vi "MotorControlMina4 with Joystick control3.vi"() -> ()   [LabVIEW 2014]
uses:
  <vilib>/Utility/inputDevices.llb/joystickAcquire.vi
  <vilib>/Utility/inputDevices.llb/closeJoystick.vi
panel:
  out "joystick info":T1(array[cluster])
  in  "Stop":bool
  out "InstrumentMode":T2(ring)=enum."Shutdown"
  in  "XMotorRef":refnum<k7>(container)
  in  "YMotorRef":refnum<k7>(container)
  in  "ZMotorRef":refnum<k7>(container)
  out "JoystOffset":T3={"XOffset"=-99999, "YOffset"=-99999, "ZOffset"=-99999}
  out "RelJoyPos":T4
  in  "InterfaceSelector":T5(tab)
  in  "GoToTopDisp":bool
  in  "GoToBottDisp":bool
  in  "GoToExpLoc":bool
  in  "SaveTopDisp":bool
  in  "SaveBottDisp":bool
  in  "SaveExpLoc":bool
  out "Top Dispenser":T6={"X Pos (mm)"=0.5532008, "Y Pos (mm)"=0.030929338, "Z Pos (mm)"=0.77973413} {"Y Pos (mm)" format="%.3f"; "Z Pos (mm)" format="%.3f"; "X Pos (mm)" format="%.3f"}
  out "Bottom Dispenser":T6={"X Pos (mm)"=0.600309, "Y Pos (mm)"=-1.1540928, "Z Pos (mm)"=0.7938141} {"Y Pos (mm)" format="%.3f"; "Z Pos (mm)" format="%.3f"; "X Pos (mm)" format="%.3f"}
  out "Experiment Region":T6={"X Pos (mm)"=1.4278219, "Y Pos (mm)"=-0.74810517, "Z Pos (mm)"=0.7938141} {"Y Pos (mm)" format="%.3f"; "Z Pos (mm)" format="%.3f"; "X Pos (mm)" format="%.3f"}
  in  "PreviewPanel":T7(tab)
  in  "Z Motor Settings":T8={"Joyst Min Signal"=10.0, "Joyst Max Signal"=30000.0, "Vmax (mm/s)"=0.005, "Acc (mm/s/s)"=0.2, "+ JoystDirection"=2, "- JoystDirection"=1} {"Acc (mm/s/s)" format="%#.3f"; "Vmax (mm/s)" format="%#.3f"}
  in  "Y Motor Settings":T8={"Joyst Min Signal"=10.0, "Joyst Max Signal"=20000.0, "Vmax (mm/s)"=0.03, "Acc (mm/s/s)"=0.5, "+ JoystDirection"=1, "- JoystDirection"=2} {"Acc (mm/s/s)" format="%#.3f"; "Vmax (mm/s)" format="%#.3f"}
  in  "X Motor Settings":T8={"Joyst Min Signal"=10.0, "Joyst Max Signal"=20000.0, "Vmax (mm/s)"=0.03, "Acc (mm/s/s)"=0.5, "+ JoystDirection"=2, "- JoystDirection"=1} {"Acc (mm/s/s)" format="%#.3f"; "Vmax (mm/s)" format="%#.3f"}
  in  "Motor Cruise Param":T9={"X Acc (mm/s^2)"=0.3, "X Vmax (mm/s)"=0.3, "Y Acc (mm/s^2)"=0.3, "Y Vmax (mm/s)"=0.3, "Z Acc (mm/s^2)"=0.1, "Z Vmax (mm/s)"=0.1}
  in  "Motor Limits":T10={"XMin"=-0.8, "XMax"=3.0, "YMin"=-2.0, "YMax"=2.0, "ZMin"=0.0, "ZMax"=2.0}
  in  "Steerable Mirror Calibration":T11={"Hor. Scaling (nm/V)"=760.0, "Vert. Scaling (nm/V)"=760.0, "Hor. Mirr. Offset (V)"=0.0, "Vert. Mirr. Offset (V)"=0.0}
  in  "Steerable \nTrap\n(F12)":bool
  in  "Fixed\nTrap\n(F11)":bool
  in  "Align Traps Vertically":bool
  in  "MaxHorizontalTrapSeparation":bool
  out "X Motor State":T12={"Direction"=0, "Vel (mm/s)"=0.0, "IsActive?"=FALSE, "Pos (mm)"=-0.2957381} {"Pos (mm)" format="%#.3f"; "Vel (mm/s)" format="%#.4f"}
  out "Y Motor State":T12={"Direction"=0, "Vel (mm/s)"=0.0, "IsActive?"=FALSE, "Pos (mm)"=0.016441232} {"Pos (mm)" format="%#.3f"; "Vel (mm/s)" format="%#.4f"}
  out "Z Motor State":T12={"Direction"=0, "Vel (mm/s)"=0.0, "IsActive?"=FALSE, "Pos (mm)"=-0.26253498} {"Pos (mm)" format="%#.3f"; "Vel (mm/s)" format="%#.4f"}
  out "Move Z":bool
  out "Move XY":bool
  in  "MotorLoopDelay":u32=100
  in  "StopPassiveMode":bool caption="stop"
  in  "PMVertSlider(V)":dbl(slide)=0.005145263671875 scale=0.0..10.0 scale format="%#_3f"
  in  "PMHorizSlider(V)":dbl(slide)=0.0045623779296875 scale=2.0..10.0
  out "IsPassiveModeActive?":bool caption="stop"
  out "Force TrapA":cluster{"x":dbl[], "y":dbl[]}[](graph)
  out "Noise-Ext":cluster{"x":dbl[], "y":dbl[]}[](graph)
  out "Force TrapB":cluster{"x":dbl[], "y":dbl[]}[](graph)
  out "IsOffsetModeActive?":bool caption="stop"
  in  "StopOffset":bool caption="stop"
  out "IsForceExtActive?":bool=TRUE
  in  "StopForceExtension":bool caption="stop"
  # "ClpXP Optical Tweezers"
  # "Chamber Locations"
  # "Need a Button Here that would read the \nNormalized Offset and save it"
  # "Off"
  # "On"
  # "Off"
  # "On"
  # "Thorlabs Motor Status"
  # "Passive Mode"
  # "when I switch tabs from the passive mode to basic mode, the recording doesn't stop"
  # "The sliders don't do anything in passive mode, fix it"
  # "Whenever I click on Ackquire Offset, it goes back to the basic operation, then I have to ckick again"
  # "Trap Motion Control"
  # "Steerable Mirror Info"
  # "Zero-Force Offset Mode"
  # "High Frequency Data Acquisition"
  # "Adjust the length of acquisition time"
  # "Force-Extension Mode"
  # "Y"
  # "+"
  # "X"
  # "-"
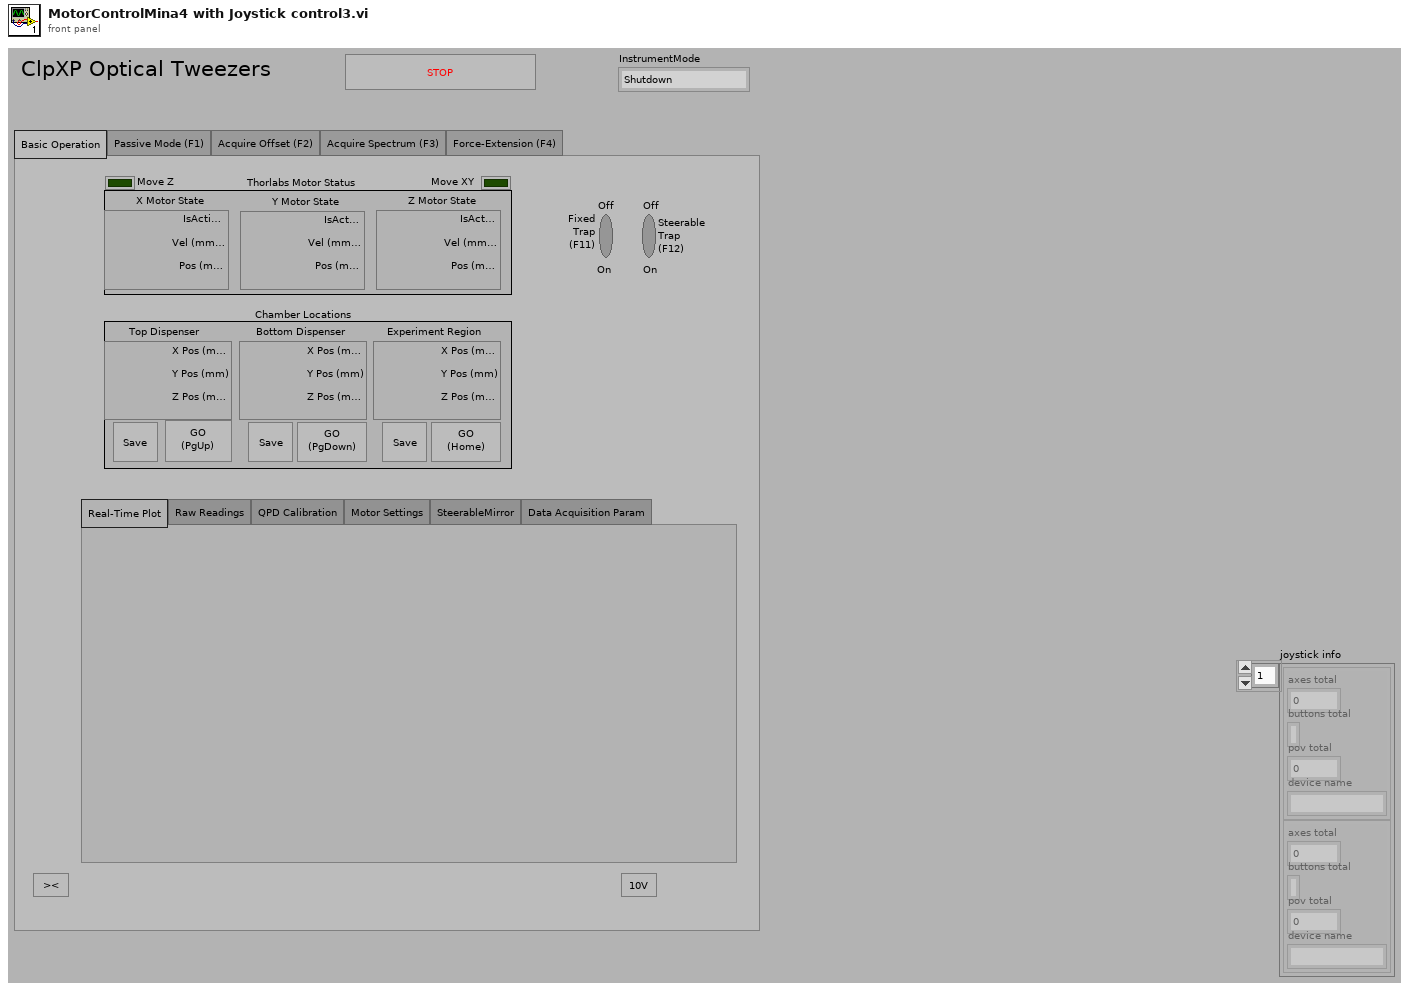
[diagram p1: front panel]
types:
  T1 = cluster{"axes total":u32, "buttons total":u32, "pov total":u32, "device name":string}[]
  T2 = enum16{"InitializeJoystick", "InitializeMotors", "BasicMode", "PassiveMode", "AcquireOffsetMode", "AcquireSpectrumMode", "Force-ExtensionMode", "Shutdown"}
  T3 = cluster{"XOffset":i32, "YOffset":i32, "ZOffset":i32}
  T4 = cluster{"XRelPos":i32, "YRelPos":i32, "ZRelPos":i32}
  T5 = enum32{"Basic Operation", "Passive Mode (F1)", "Acquire Offset (F2)", "Acquire Spectrum (F3)", "Force-Extension (F4)"}
  T6 = cluster{"X Pos (mm)":sgl, "Y Pos (mm)":sgl, "Z Pos (mm)":sgl}
  T7 = enum32{"Real-Time Plot", "Raw Readings", "QPD Calibration", "Motor Settings", "SteerableMirror", "Data Acquisition Param"}
  T8 = cluster{"Joyst Min Signal":dbl, "Joyst Max Signal":dbl, "Vmax (mm/s)":sgl, "Acc (mm/s/s)":sgl, "+ JoystDirection":i32, "- JoystDirection":i32}
  T9 = cluster{"X Acc (mm/s^2)":sgl, "X Vmax (mm/s)":sgl, "Y Acc (mm/s^2)":sgl, "Y Vmax (mm/s)":sgl, "Z Acc (mm/s^2)":sgl, "Z Vmax (mm/s)":sgl}
  T10 = cluster{"XMin":sgl, "XMax":sgl, "YMin":sgl, "YMax":sgl, "ZMin":sgl, "ZMax":sgl}
  T11 = cluster{"Hor. Scaling (nm/V)":dbl, "Vert. Scaling (nm/V)":dbl, "Hor. Mirr. Offset (V)":dbl, "Vert. Mirr. Offset (V)":dbl}
  T12 = cluster{"Direction":i32, "Vel (mm/s)":sgl, "IsActive?":bool, "Pos (mm)":sgl}
  T13 = cluster{"XMotorRef":refnum<k7>, "YMotorRef":refnum<k7>, "ZMotorRef":refnum<k7>}
  T14 = cluster{"Motor Reference":refnum<k7>, "Motor Reference":refnum<k7>, "Motor Reference":refnum<k7>}
  T15 = cluster{"X axis":i32, "Y axis":i32, "Z axis":i32, "X axis rotation":i32, "Y axis rotation":i32, "Z axis rotation":i32, "U axis":i32, "V axis":i32}
  T16 = cluster{"button 1":bool, "button 2":bool, "button 3":bool, "button 4":bool, "button 5":bool, "button 6":bool, "button 7":bool, "button 8":bool, "button 9":bool, "button 10":bool, "button 11":bool, "button 12":bool, "button 13":bool, "button 14":bool, "button 15":bool, "button 16":bool, "button 17":bool, "button 18":bool, "button 19":bool, "button 20":bool, "button 21":bool, "button 22":bool, "button 23":bool, "button 24":bool, "button 25":bool, "button 26":bool, "button 27":bool, "button 28":bool, "button 29":bool, "button 30":bool, "button 31":bool, "button 32":bool}
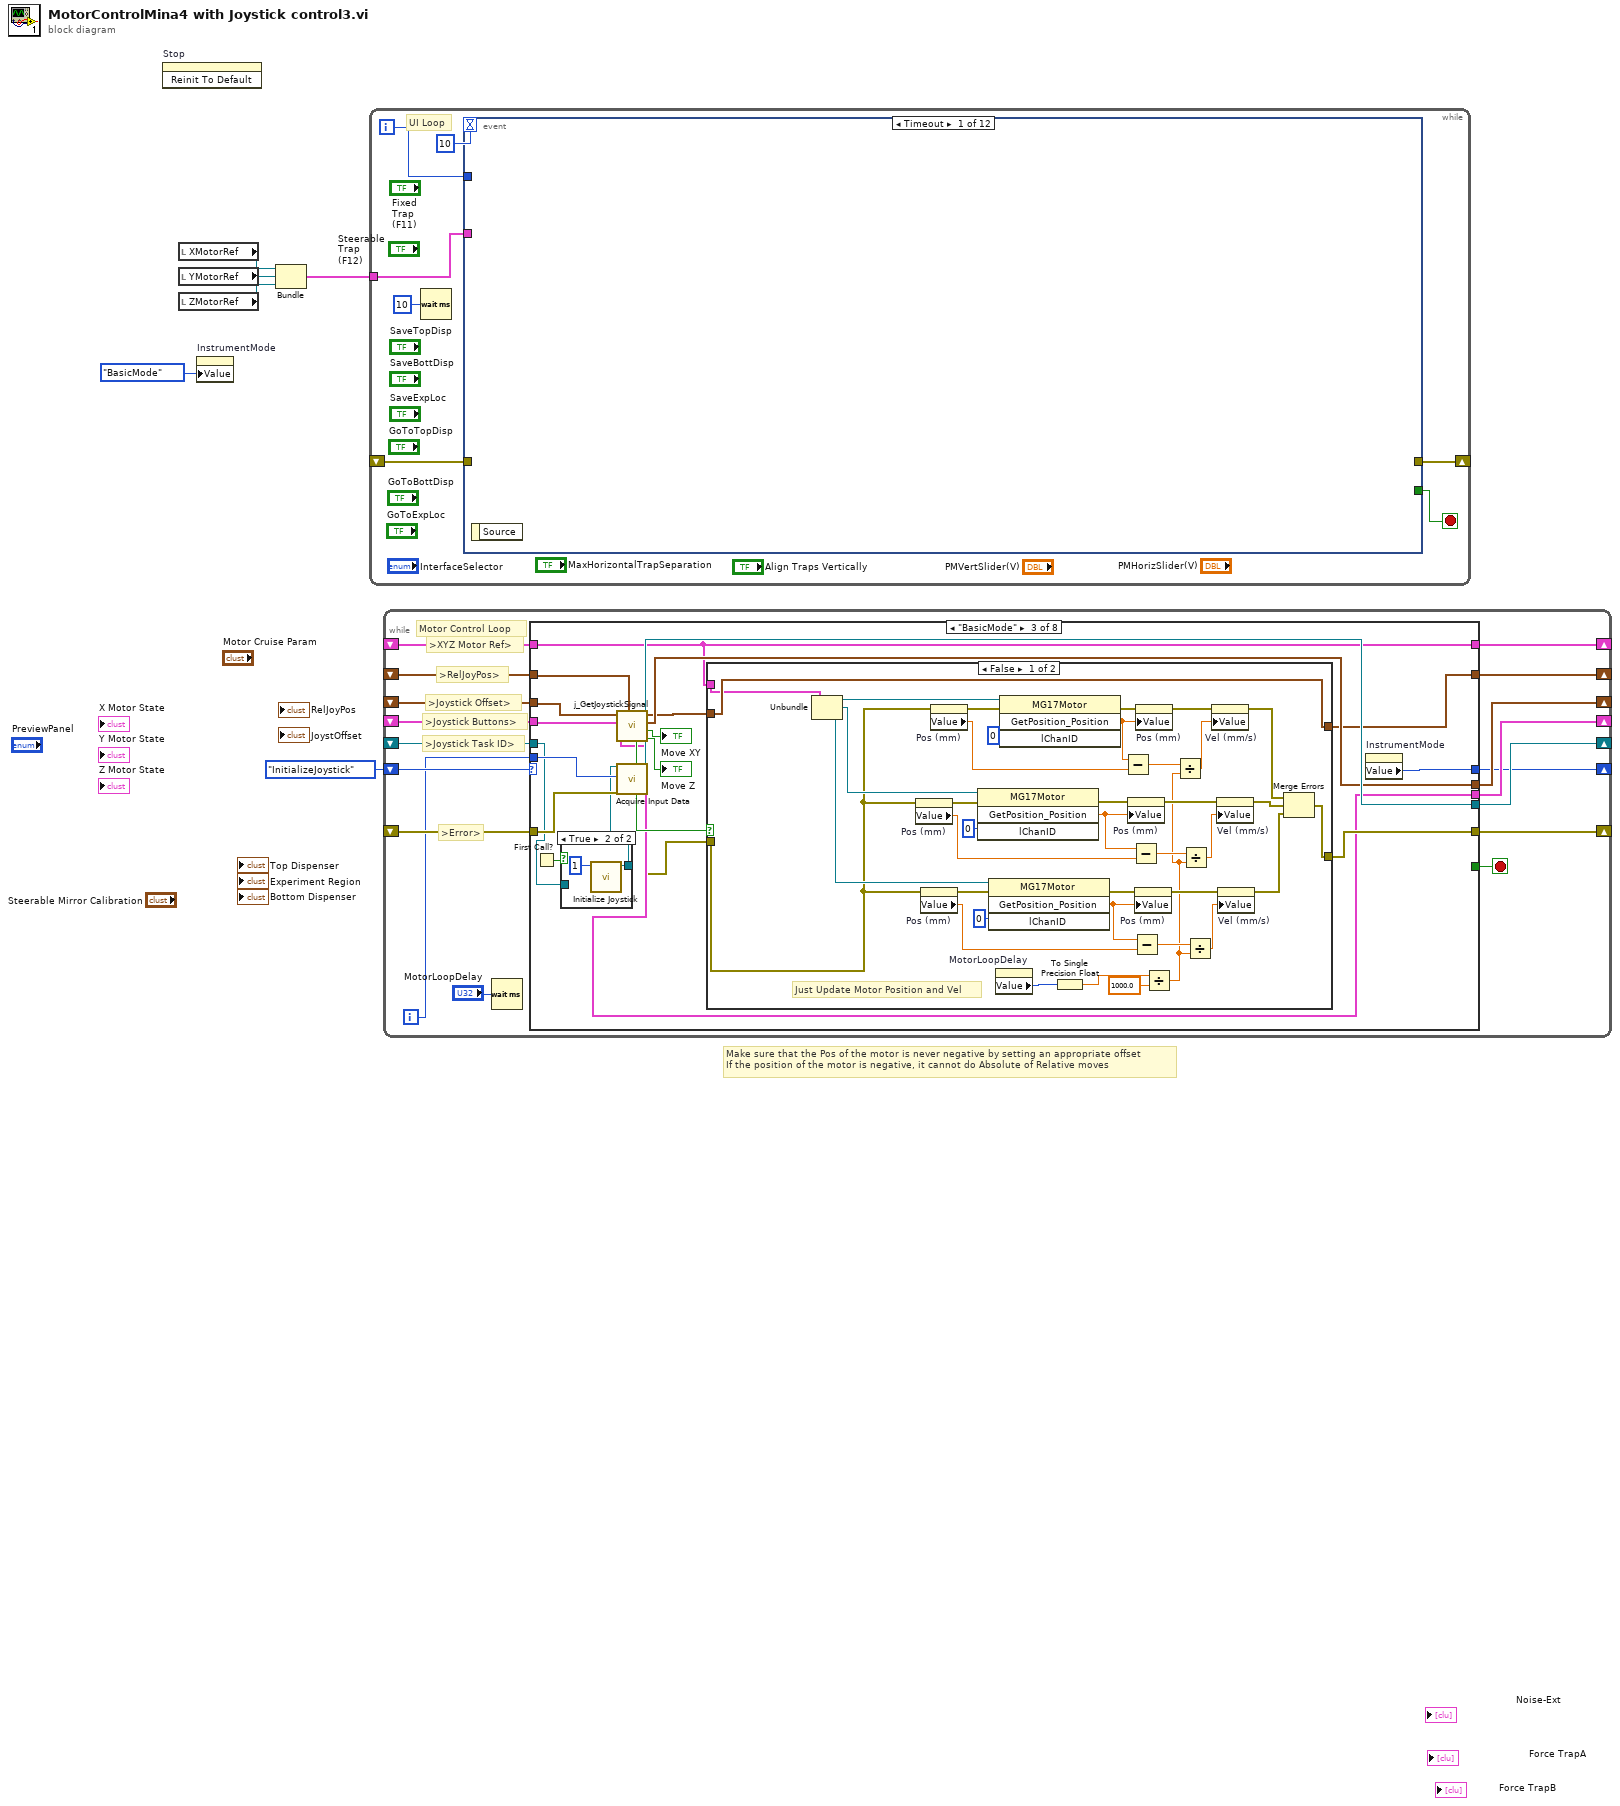
[diagram p0: block diagram]
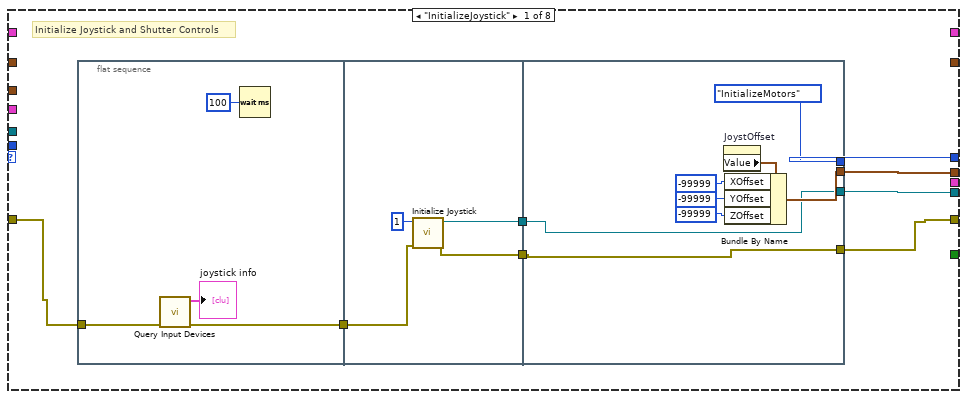
[diagram p2: hidden frame]
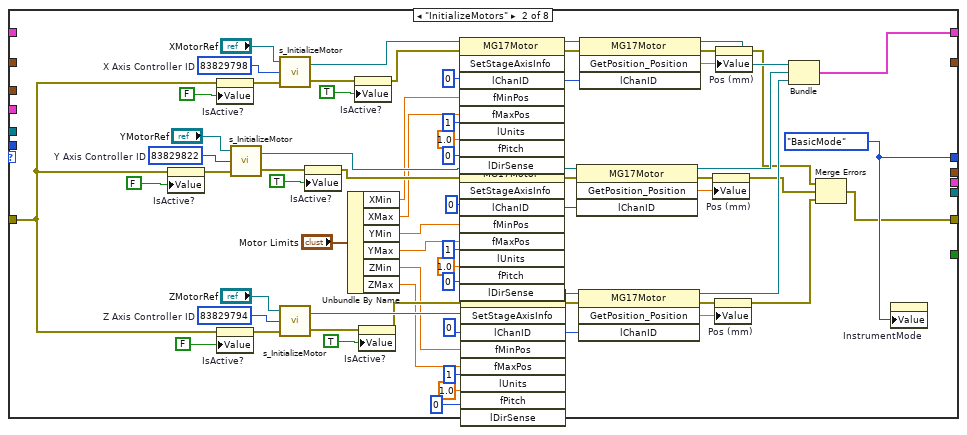
[diagram p3: hidden frame]
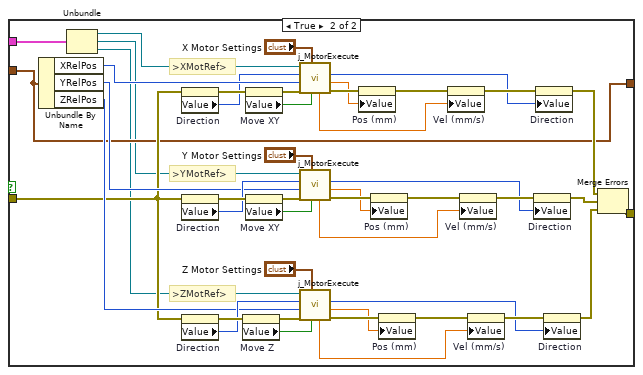
[diagram p5: hidden frame]
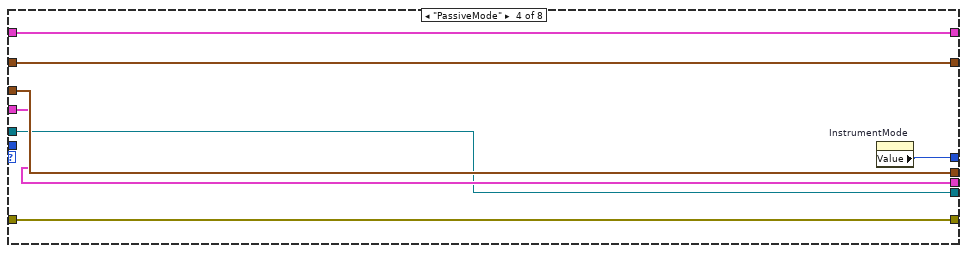
[diagram p6: hidden frame]
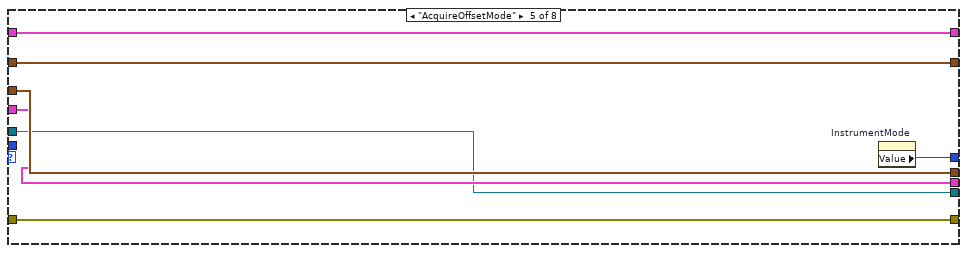
[diagram p7: hidden frame]
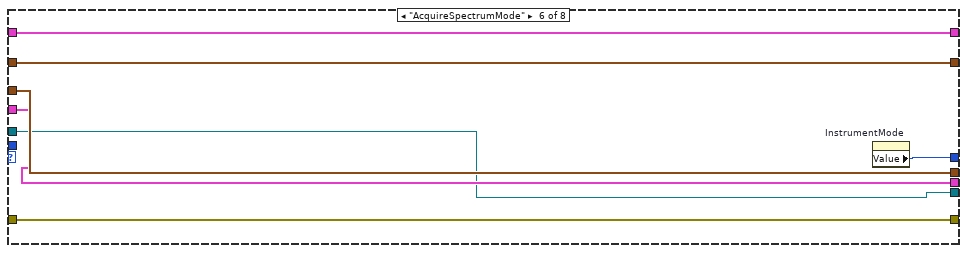
[diagram p8: hidden frame]
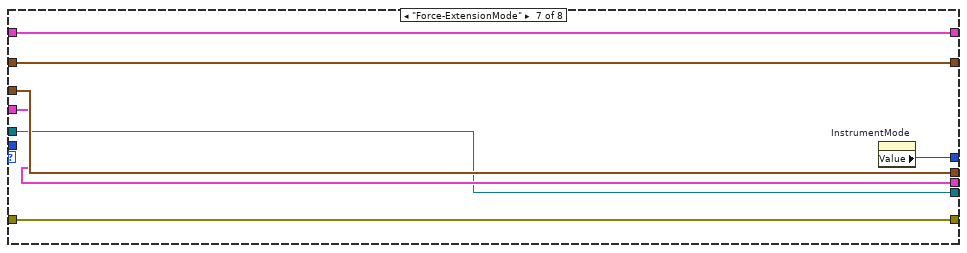
[diagram p9: hidden frame]
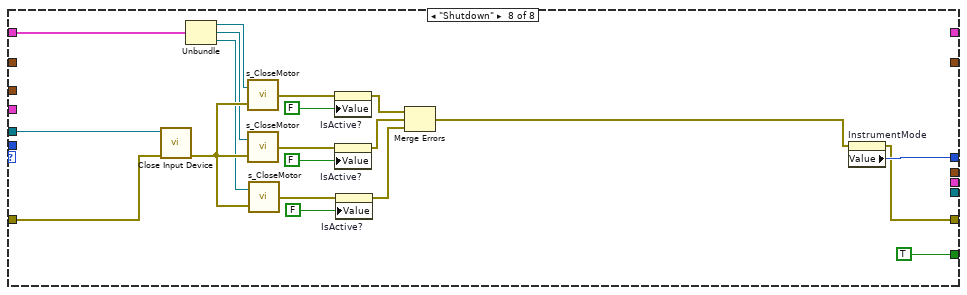
[diagram p10: hidden frame]
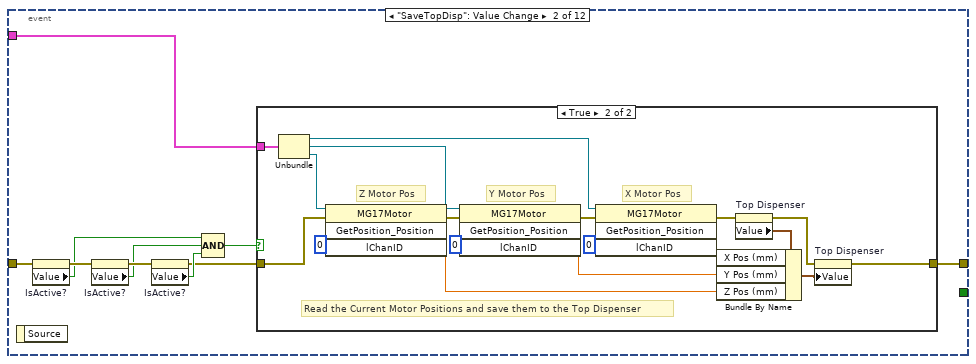
[diagram p11: hidden frame]
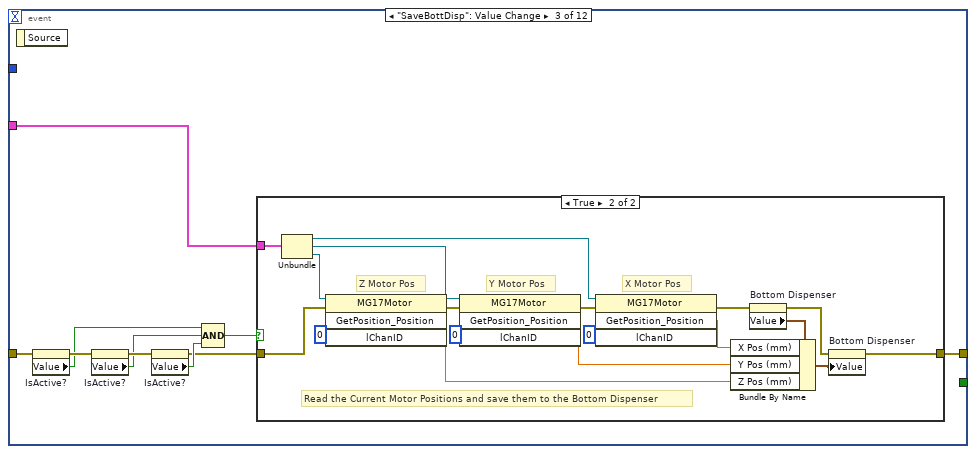
[diagram p13: hidden frame]
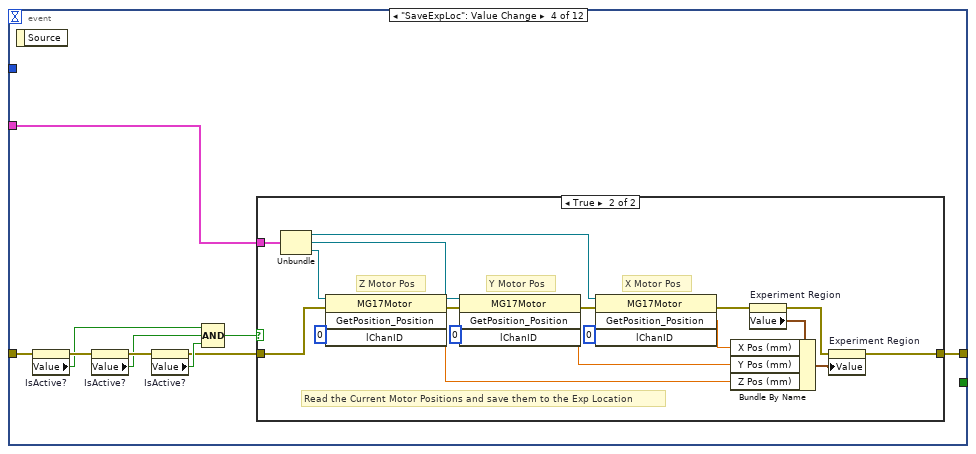
[diagram p15: hidden frame]
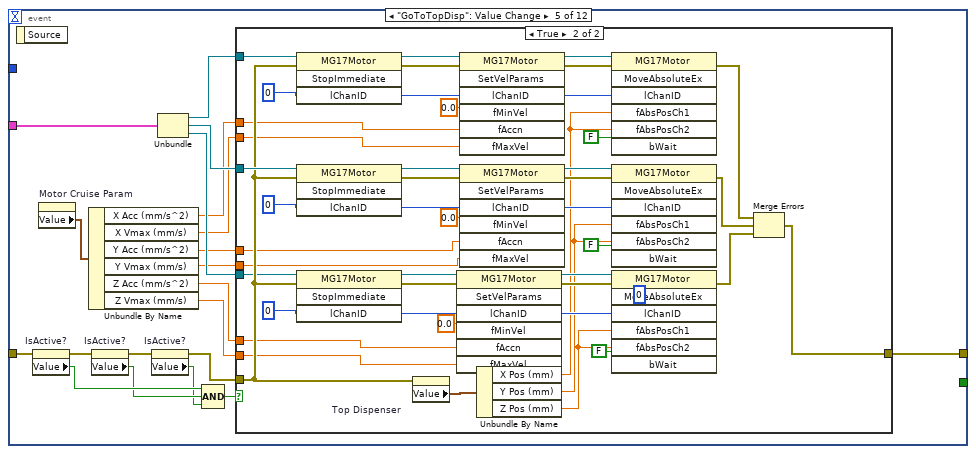
[diagram p17: hidden frame]
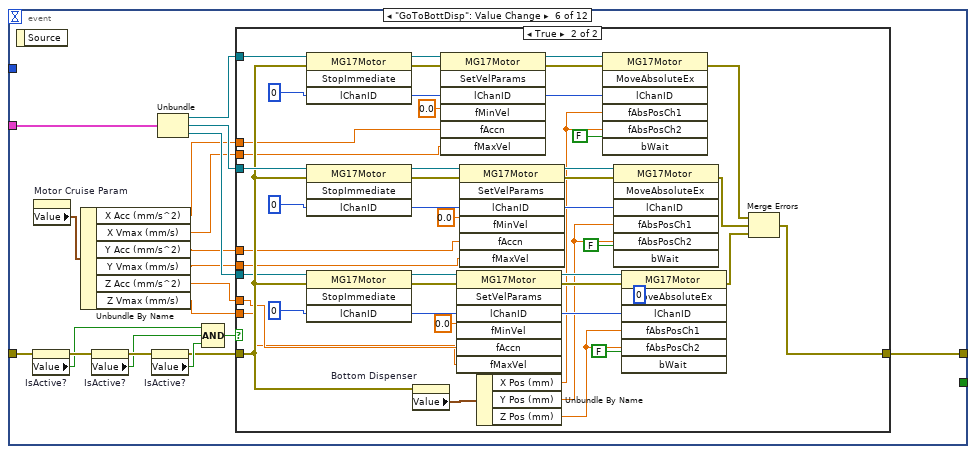
[diagram p19: hidden frame]
diagram:
  # "Make sure that the Pos of the motor is never negative by setting an appropriate offset\nIf the position of the motor is negative, it cannot do Absolute of Relative moves"
  n1 = invoke on="Stop" class="Bool" method="Reinit To Default"() -> ()  [unwired: 3 in, 3 out]
  n2 = local read "XMotorRef"() -> (w6:refnum<k7>)
  n3 = local read "YMotorRef"() -> (w5:refnum<k7>)
  n4 = local read "ZMotorRef"() -> (w4:refnum<k7>)
  n5 = property on="InstrumentMode" class="Enum (strict)"("Value"=T2."BasicMode") -> ()  [unwired: 2 in, 2 out]
  n6 = Bundle("XMotorRef"=w6, "YMotorRef"=w5, "ZMotorRef"=w4) -> (w3:T13)  [unwired: 1 in]
  n7 = while {
    shift-right: [w12] -> _
    shift-left: _ -> [w11]
    tunnel: w3 -> [w10]
    i -> [w8]
    stop <- w9 stop-if-true
    # "UI Loop"
    n8 = Wait (ms)(milliseconds to wait=u32 10) -> ()  [unwired: 1 out]
    n9 = event shown="[0] Timeout" {
      selector: _ -> [_ _ _ _ _ _ _ _ _ _ _ _]
      dyn-events: _ -> [_ _ _ _ _ _ _ _ _ _ _ _]
      timeout: 10 -> [_ _ _ _ _ _ _ _ _ _ _ _]
      tunnel: [_ w16 w45 w74 w113 w179 w245 w299 _ _ _ w327] -> w12
      tunnel: w11 -> [_ w15 w44 w73 w112 w178 w244 w299 _ _ _ w327]
      tunnel: [_ _ _ _ _ _ _ _ _ _ _ "Stop"] -> w9
      tunnel: w10 -> [_ w14 w43 w72 w111 w177 w243 _ _ _ _ _]
      tunnel: w8 -> [_ _ _ _ _ _ _ _ _ _ _ _]
      event Timeout {
        n10 = event-data() -> ()  [unwired: 1 in, 1 out]
      }
      event "SaveTopDisp": Value Change {
        n11 = event-data() -> ()  [unwired: 1 in, 1 out]
        n12 = property on="IsActive?" class="Bool (strict)"(error in=w15) -> (error out=w23:errorcluster, "Value"=w21:bool)  [unwired: 1 in, 1 out]
        n13 = property on="IsActive?" class="Bool (strict)"(error in=w23) -> (error out=w22:errorcluster, "Value"=w20:bool)  [unwired: 1 in, 1 out]
        n14 = property on="IsActive?" class="Bool (strict)"(error in=w22) -> (error out=w17:errorcluster, "Value"=w19:bool)  [unwired: 1 in, 1 out]
        n15 = Compound Arithmetic op=AND(w21, w20, w19) -> (w18:bool)
        n16 = case shown="True" w18 {
          tunnel: w17 -> [w24 w42]
          tunnel: [w24 w29] -> w16
          tunnel: w14 -> [_ w28]
          frame False {
          }
          frame True {
            # "Read the Current Motor Positions and save them to the Top Dispenser"
            # "X Motor Pos"
            # "Y Motor Pos"
            # "Z Motor Pos"
            n17 = Unbundle(w28) -> ("XMotorRef"=w25:refnum<k7>, "YMotorRef"=w26:refnum<k7>, "ZMotorRef"=w27:refnum<k7>)
            n18 = invoke class="MG17Motor" method="GetPosition_Position"(reference=w27, error in=w42, "lChanID"=0) -> (error out=w39:errorcluster, "GetPosition_Position"=w32:sgl)  [unwired: 1 in, 2 out]
            n19 = invoke class="MG17Motor" method="GetPosition_Position"(reference=w26, error in=w39, "lChanID"=0) -> (error out=w37:errorcluster, "GetPosition_Position"=w31:sgl)  [unwired: 1 in, 2 out]
            n20 = invoke class="MG17Motor" method="GetPosition_Position"(reference=w25, error in=w37, "lChanID"=0) -> (error out=w36:errorcluster, "GetPosition_Position"=w30:sgl)  [unwired: 1 in, 2 out]
            n21 = property on="Top Dispenser" class="Clust (strict)"(error in=w36) -> (error out=w35:errorcluster, "Value"=w34:T6)  [unwired: 1 in, 1 out]
            n22 = Bundle By Name(cluster=w34, "X Pos (mm)"=w30, "Y Pos (mm)"=w31, "Z Pos (mm)"=w32) -> (w33:T6)
            n23 = property on="Top Dispenser" class="Clust (strict)"(error in=w35, "Value"=w33) -> (error out=w29:errorcluster)  [unwired: 1 in, 1 out]
          }
        }
      }
      event "SaveBottDisp": Value Change {
        n24 = event-data() -> ()  [unwired: 1 in, 1 out]
        n25 = property on="IsActive?" class="Bool (strict)"(error in=w44) -> (error out=w52:errorcluster, "Value"=w50:bool)  [unwired: 1 in, 1 out]
        n26 = property on="IsActive?" class="Bool (strict)"(error in=w52) -> (error out=w51:errorcluster, "Value"=w49:bool)  [unwired: 1 in, 1 out]
        n27 = property on="IsActive?" class="Bool (strict)"(error in=w51) -> (error out=w46:errorcluster, "Value"=w48:bool)  [unwired: 1 in, 1 out]
        n28 = Compound Arithmetic op=AND(w50, w49, w48) -> (w47:bool)
        n29 = case shown="True" w47 {
          tunnel: w46 -> [w53 w71]
          tunnel: [w53 w58] -> w45
          tunnel: w43 -> [_ w57]
          frame False {
          }
          frame True {
            # "Read the Current Motor Positions and save them to the Bottom Dispenser"
            # "X Motor Pos"
            # "Y Motor Pos"
            # "Z Motor Pos"
            n30 = Unbundle(w57) -> ("XMotorRef"=w54:refnum<k7>, "YMotorRef"=w55:refnum<k7>, "ZMotorRef"=w56:refnum<k7>)
            n31 = invoke class="MG17Motor" method="GetPosition_Position"(reference=w56, error in=w71, "lChanID"=0) -> (error out=w68:errorcluster, "GetPosition_Position"=w61:sgl)  [unwired: 1 in, 2 out]
            n32 = invoke class="MG17Motor" method="GetPosition_Position"(reference=w55, error in=w68, "lChanID"=0) -> (error out=w66:errorcluster, "GetPosition_Position"=w60:sgl)  [unwired: 1 in, 2 out]
            n33 = invoke class="MG17Motor" method="GetPosition_Position"(reference=w54, error in=w66, "lChanID"=0) -> (error out=w65:errorcluster, "GetPosition_Position"=w59:sgl)  [unwired: 1 in, 2 out]
            n34 = property on="Bottom Dispenser" class="Clust (strict)"(error in=w65) -> (error out=w64:errorcluster, "Value"=w63:T6)  [unwired: 1 in, 1 out]
            n35 = Bundle By Name(cluster=w63, "X Pos (mm)"=w59, "Y Pos (mm)"=w60, "Z Pos (mm)"=w61) -> (w62:T6)
            n36 = property on="Bottom Dispenser" class="Clust (strict)"(error in=w64, "Value"=w62) -> (error out=w58:errorcluster)  [unwired: 1 in, 1 out]
          }
        }
      }
      event "SaveExpLoc": Value Change {
        n37 = event-data() -> ()  [unwired: 1 in, 1 out]
        n38 = property on="IsActive?" class="Bool (strict)"(error in=w73) -> (error out=w81:errorcluster, "Value"=w79:bool)  [unwired: 1 in, 1 out]
        n39 = property on="IsActive?" class="Bool (strict)"(error in=w81) -> (error out=w80:errorcluster, "Value"=w78:bool)  [unwired: 1 in, 1 out]
        n40 = property on="IsActive?" class="Bool (strict)"(error in=w80) -> (error out=w75:errorcluster, "Value"=w77:bool)  [unwired: 1 in, 1 out]
        n41 = Compound Arithmetic op=AND(w79, w78, w77) -> (w76:bool)
        n42 = case shown="True" w76 {
          tunnel: w75 -> [w82 w100]
          tunnel: [w82 w87] -> w74
          tunnel: w72 -> [_ w86]
          frame False {
          }
          frame True {
            # "Read the Current Motor Positions and save them to the Exp Location"
            # "X Motor Pos"
            # "Y Motor Pos"
            # "Z Motor Pos"
            n43 = Unbundle(w86) -> ("XMotorRef"=w83:refnum<k7>, "YMotorRef"=w84:refnum<k7>, "ZMotorRef"=w85:refnum<k7>)
            n44 = invoke class="MG17Motor" method="GetPosition_Position"(reference=w85, error in=w100, "lChanID"=0) -> (error out=w97:errorcluster, "GetPosition_Position"=w90:sgl)  [unwired: 1 in, 2 out]
            n45 = invoke class="MG17Motor" method="GetPosition_Position"(reference=w84, error in=w97, "lChanID"=0) -> (error out=w95:errorcluster, "GetPosition_Position"=w89:sgl)  [unwired: 1 in, 2 out]
            n46 = invoke class="MG17Motor" method="GetPosition_Position"(reference=w83, error in=w95, "lChanID"=0) -> (error out=w94:errorcluster, "GetPosition_Position"=w88:sgl)  [unwired: 1 in, 2 out]
            n47 = property on="Experiment Region" class="Clust (strict)"(error in=w94) -> (error out=w93:errorcluster, "Value"=w92:T6)  [unwired: 1 in, 1 out]
            n48 = Bundle By Name(cluster=w92, "X Pos (mm)"=w88, "Y Pos (mm)"=w89, "Z Pos (mm)"=w90) -> (w91:T6)
            n49 = property on="Experiment Region" class="Clust (strict)"(error in=w93, "Value"=w91) -> (error out=w87:errorcluster)  [unwired: 1 in, 1 out]
          }
        }
      }
      event "GoToTopDisp": Value Change {
        n50 = event-data() -> ()  [unwired: 1 in, 1 out]
        n51 = property on="IsActive?" class="Bool (strict)"(error in=w112) -> (error out=w120:errorcluster, "Value"=w118:bool)  [unwired: 1 in, 1 out]
        n52 = property on="Motor Cruise Param" class="Clust (strict)"() -> ("Value"=w101:T9)  [unwired: 2 in, 2 out]
        n53 = Unbundle By Name(w101) -> ("X Acc (mm/s^2)"=w105:sgl, "X Vmax (mm/s)"=w104:sgl, "Y Acc (mm/s^2)"=w103:sgl, "Y Vmax (mm/s)"=w102:sgl, "Z Acc (mm/s^2)"=w107:sgl, "Z Vmax (mm/s)"=w106:sgl)
        n54 = property on="IsActive?" class="Bool (strict)"(error in=w120) -> (error out=w119:errorcluster, "Value"=w117:bool)  [unwired: 1 in, 1 out]
        n55 = property on="IsActive?" class="Bool (strict)"(error in=w119) -> (error out=w114:errorcluster, "Value"=w116:bool)  [unwired: 1 in, 1 out]
        n56 = Unbundle(w111) -> ("XMotorRef"=w110:refnum<k7>, "YMotorRef"=w109:refnum<k7>, "ZMotorRef"=w108:refnum<k7>)
        n57 = Compound Arithmetic op=AND(w118, w117, w116) -> (w115:bool)
        n58 = case shown="True" w115 {
          tunnel: w114 -> [w121 w141]
          tunnel: [w121 w137] -> w113
          tunnel: w110 -> [_ w164]
          tunnel: w109 -> [_ w149]
          tunnel: w108 -> [_ w136]
          tunnel: w107 -> [_ w127]
          tunnel: w106 -> [_ w126]
          tunnel: w105 -> [_ w125]
          tunnel: w104 -> [_ w124]
          tunnel: w103 -> [_ w123]
          tunnel: w102 -> [_ w122]
          frame False {
          }
          frame True {
            (unwired) 0 ("lChanID")
            n59 = invoke class="MG17Motor" method="StopImmediate"(reference=w164, error in=w141, "lChanID"=0) -> (reference out=w162:refnum<k7>, error out=w163:errorcluster, "lChanID"=w132:i32)  [unwired: 1 in, 1 out]
            n60 = invoke class="MG17Motor" method="StopImmediate"(reference=w149, error in=w141, "lChanID"=0) -> (reference out=w156:refnum<k7>, error out=w157:errorcluster, "lChanID"=w133:i32)  [unwired: 1 in, 1 out]
            n61 = invoke class="MG17Motor" method="StopImmediate"(reference=w136, error in=w141, "lChanID"=0) -> (reference out=w146:refnum<k7>, error out=w147:errorcluster, "lChanID"=w134:i32)  [unwired: 1 in, 1 out]
            n62 = property on="Top Dispenser" class="Clust (strict)"(error in=w141) -> ("Value"=w166:T6)  [unwired: 1 in, 2 out]
            n63 = invoke class="MG17Motor" method="SetVelParams"(reference=w146, error in=w147, "lChanID"=w134, "fMinVel"=sgl 0.0, "fAccn"=w127, "fMaxVel"=w126) -> (reference out=w145:refnum<k7>, error out=w144:errorcluster, "lChanID"=w143:i32)  [unwired: 1 in, 4 out]
            n64 = invoke class="MG17Motor" method="SetVelParams"(reference=w162, error in=w163, "lChanID"=w132, "fMinVel"=sgl 0.0, "fAccn"=w125, "fMaxVel"=w124) -> (reference out=w161:refnum<k7>, error out=w160:errorcluster, "lChanID"=w159:i32)  [unwired: 1 in, 4 out]
            n65 = invoke class="MG17Motor" method="SetVelParams"(reference=w156, error in=w157, "lChanID"=w133, "fMinVel"=sgl 0.0, "fAccn"=w123, "fMaxVel"=w122) -> (reference out=w154:refnum<k7>, error out=w153:errorcluster, "lChanID"=w152:i32)  [unwired: 1 in, 4 out]
            n66 = Unbundle By Name(w166) -> ("X Pos (mm)"=w130:sgl, "Y Pos (mm)"=w129:sgl, "Z Pos (mm)"=w128:sgl)
            n67 = invoke class="MG17Motor" method="MoveAbsoluteEx"(reference=w161, error in=w160, "lChanID"=w159, "fAbsPosCh1"=w130, "fAbsPosCh2"=w130, "bWait"=FALSE) -> (error out=w140:errorcluster)  [unwired: 1 in, 6 out]
            n68 = invoke class="MG17Motor" method="MoveAbsoluteEx"(reference=w154, error in=w153, "lChanID"=w152, "fAbsPosCh1"=w129, "fAbsPosCh2"=w129, "bWait"=FALSE) -> (error out=w139:errorcluster)  [unwired: 1 in, 6 out]
            n69 = invoke class="MG17Motor" method="MoveAbsoluteEx"(reference=w145, error in=w144, "lChanID"=w143, "fAbsPosCh1"=w128, "fAbsPosCh2"=w128, "bWait"=FALSE) -> (error out=w138:errorcluster)  [unwired: 1 in, 6 out]
            n70 = Merge Errors(w140, w139, w138) -> (w137:errorcluster)
          }
        }
      }
      event "GoToBottDisp": Value Change {
        n71 = event-data() -> ()  [unwired: 1 in, 1 out]
        n72 = property on="IsActive?" class="Bool (strict)"(error in=w178) -> (error out=w186:errorcluster, "Value"=w184:bool)  [unwired: 1 in, 1 out]
        n73 = property on="Motor Cruise Param" class="Clust (strict)"() -> ("Value"=w173:T9)  [unwired: 2 in, 2 out]
        n74 = Unbundle By Name(w173) -> ("X Acc (mm/s^2)"=w172:sgl, "X Vmax (mm/s)"=w171:sgl, "Y Acc (mm/s^2)"=w170:sgl, "Y Vmax (mm/s)"=w169:sgl, "Z Acc (mm/s^2)"=w168:sgl, "Z Vmax (mm/s)"=w167:sgl)
        n75 = property on="IsActive?" class="Bool (strict)"(error in=w186) -> (error out=w185:errorcluster, "Value"=w183:bool)  [unwired: 1 in, 1 out]
        n76 = property on="IsActive?" class="Bool (strict)"(error in=w185) -> (error out=w180:errorcluster, "Value"=w182:bool)  [unwired: 1 in, 1 out]
        n77 = Unbundle(w177) -> ("XMotorRef"=w176:refnum<k7>, "YMotorRef"=w175:refnum<k7>, "ZMotorRef"=w174:refnum<k7>)
        n78 = Compound Arithmetic op=AND(w184, w183, w182) -> (w181:bool)
        n79 = case shown="True" w181 {
          tunnel: w180 -> [w187 w207]
          tunnel: [w187 w203] -> w179
          tunnel: w176 -> [_ w230]
          tunnel: w175 -> [_ w215]
          tunnel: w174 -> [_ w202]
          tunnel: w172 -> [_ w193]
          tunnel: w171 -> [_ w192]
          tunnel: w170 -> [_ w191]
          tunnel: w169 -> [_ w190]
          tunnel: w168 -> [_ w189]
          tunnel: w167 -> [_ w188]
          frame False {
          }
          frame True {
            (unwired) 0 ("lChanID")
            n80 = invoke class="MG17Motor" method="StopImmediate"(reference=w230, error in=w207, "lChanID"=0) -> (reference out=w228:refnum<k7>, error out=w229:errorcluster, "lChanID"=w198:i32)  [unwired: 1 in, 1 out]
            n81 = invoke class="MG17Motor" method="StopImmediate"(reference=w215, error in=w207, "lChanID"=0) -> (reference out=w222:refnum<k7>, error out=w223:errorcluster, "lChanID"=w199:i32)  [unwired: 1 in, 1 out]
            n82 = invoke class="MG17Motor" method="StopImmediate"(reference=w202, error in=w207, "lChanID"=0) -> (reference out=w212:refnum<k7>, error out=w213:errorcluster, "lChanID"=w200:i32)  [unwired: 1 in, 1 out]
            n83 = property on="Bottom Dispenser" class="Clust (strict)"(error in=w207) -> ("Value"=w232:T6)  [unwired: 1 in, 2 out]
            n84 = invoke class="MG17Motor" method="SetVelParams"(reference=w228, error in=w229, "lChanID"=w198, "fMinVel"=sgl 0.0, "fAccn"=w193, "fMaxVel"=w192) -> (reference out=w227:refnum<k7>, error out=w226:errorcluster, "lChanID"=w225:i32)  [unwired: 1 in, 4 out]
            n85 = invoke class="MG17Motor" method="SetVelParams"(reference=w212, error in=w213, "lChanID"=w200, "fMinVel"=sgl 0.0, "fAccn"=w189, "fMaxVel"=w188) -> (reference out=w211:refnum<k7>, error out=w210:errorcluster, "lChanID"=w209:i32)  [unwired: 1 in, 4 out]
            n86 = invoke class="MG17Motor" method="SetVelParams"(reference=w222, error in=w223, "lChanID"=w199, "fMinVel"=sgl 0.0, "fAccn"=w191, "fMaxVel"=w190) -> (reference out=w220:refnum<k7>, error out=w219:errorcluster, "lChanID"=w218:i32)  [unwired: 1 in, 4 out]
            n87 = Unbundle By Name(w232) -> ("X Pos (mm)"=w196:sgl, "Y Pos (mm)"=w195:sgl, "Z Pos (mm)"=w194:sgl)
            n88 = invoke class="MG17Motor" method="MoveAbsoluteEx"(reference=w227, error in=w226, "lChanID"=w225, "fAbsPosCh1"=w196, "fAbsPosCh2"=w196, "bWait"=FALSE) -> (error out=w206:errorcluster)  [unwired: 1 in, 6 out]
            n89 = invoke class="MG17Motor" method="MoveAbsoluteEx"(reference=w220, error in=w219, "lChanID"=w218, "fAbsPosCh1"=w195, "fAbsPosCh2"=w195, "bWait"=FALSE) -> (error out=w205:errorcluster)  [unwired: 1 in, 6 out]
            n90 = invoke class="MG17Motor" method="MoveAbsoluteEx"(reference=w211, error in=w210, "lChanID"=w209, "fAbsPosCh1"=w194, "fAbsPosCh2"=w194, "bWait"=FALSE) -> (error out=w204:errorcluster)  [unwired: 1 in, 6 out]
            n91 = Merge Errors(w206, w205, w204) -> (w203:errorcluster)
          }
        }
      }
      event "GoToExpLoc": Value Change {
        n92 = event-data() -> ()  [unwired: 1 in, 1 out]
        n93 = property on="Motor Cruise Param" class="Clust (strict)"() -> ("Value"=w239:T9)  [unwired: 2 in, 2 out]
        n94 = property on="IsActive?" class="Bool (strict)"(error in=w244) -> (error out=w252:errorcluster, "Value"=w250:bool)  [unwired: 1 in, 1 out]
        n95 = Unbundle By Name(w239) -> ("X Acc (mm/s^2)"=w238:sgl, "X Vmax (mm/s)"=w237:sgl, "Y Acc (mm/s^2)"=w236:sgl, "Y Vmax (mm/s)"=w235:sgl, "Z Acc (mm/s^2)"=w234:sgl, "Z Vmax (mm/s)"=w233:sgl)
        n96 = property on="IsActive?" class="Bool (strict)"(error in=w252) -> (error out=w251:errorcluster, "Value"=w249:bool)  [unwired: 1 in, 1 out]
        n97 = property on="IsActive?" class="Bool (strict)"(error in=w251) -> (error out=w246:errorcluster, "Value"=w248:bool)  [unwired: 1 in, 1 out]
        n98 = Unbundle(w243) -> ("XMotorRef"=w242:refnum<k7>, "YMotorRef"=w241:refnum<k7>, "ZMotorRef"=w240:refnum<k7>)
        n99 = Compound Arithmetic op=AND(w250, w249, w248) -> (w247:bool)
        n100 = case shown="True" w247 {
          tunnel: w246 -> [w253 w273]
          tunnel: [w253 w269] -> w245
          tunnel: w242 -> [_ w296]
          tunnel: w241 -> [_ w281]
          tunnel: w240 -> [_ w268]
          tunnel: w238 -> [_ w259]
          tunnel: w237 -> [_ w258]
          tunnel: w236 -> [_ w257]
          tunnel: w235 -> [_ w256]
          tunnel: w234 -> [_ w255]
          tunnel: w233 -> [_ w254]
          frame False {
          }
          frame True {
            (unwired) 0 ("lChanID")
            n101 = invoke class="MG17Motor" method="StopImmediate"(reference=w296, error in=w273, "lChanID"=0) -> (reference out=w294:refnum<k7>, error out=w295:errorcluster, "lChanID"=w264:i32)  [unwired: 1 in, 1 out]
            n102 = invoke class="MG17Motor" method="StopImmediate"(reference=w281, error in=w273, "lChanID"=0) -> (reference out=w288:refnum<k7>, error out=w289:errorcluster, "lChanID"=w265:i32)  [unwired: 1 in, 1 out]
            n103 = invoke class="MG17Motor" method="StopImmediate"(reference=w268, error in=w273, "lChanID"=0) -> (reference out=w278:refnum<k7>, error out=w279:errorcluster, "lChanID"=w266:i32)  [unwired: 1 in, 1 out]
            n104 = property on="Experiment Region" class="Clust (strict)"(error in=w273) -> ("Value"=w298:T6)  [unwired: 1 in, 2 out]
            n105 = invoke class="MG17Motor" method="SetVelParams"(reference=w294, error in=w295, "lChanID"=w264, "fMinVel"=sgl 0.0, "fAccn"=w259, "fMaxVel"=w258) -> (reference out=w293:refnum<k7>, error out=w292:errorcluster, "lChanID"=w291:i32)  [unwired: 1 in, 4 out]
            n106 = invoke class="MG17Motor" method="SetVelParams"(reference=w278, error in=w279, "lChanID"=w266, "fMinVel"=sgl 0.0, "fAccn"=w255, "fMaxVel"=w254) -> (reference out=w277:refnum<k7>, error out=w276:errorcluster, "lChanID"=w275:i32)  [unwired: 1 in, 4 out]
            n107 = invoke class="MG17Motor" method="SetVelParams"(reference=w288, error in=w289, "lChanID"=w265, "fMinVel"=sgl 0.0, "fAccn"=w257, "fMaxVel"=w256) -> (reference out=w286:refnum<k7>, error out=w285:errorcluster, "lChanID"=w284:i32)  [unwired: 1 in, 4 out]
            n108 = Unbundle By Name(w298) -> ("X Pos (mm)"=w262:sgl, "Y Pos (mm)"=w261:sgl, "Z Pos (mm)"=w260:sgl)
            n109 = invoke class="MG17Motor" method="MoveAbsoluteEx"(reference=w293, error in=w292, "lChanID"=w291, "fAbsPosCh1"=w262, "fAbsPosCh2"=w262, "bWait"=FALSE) -> (error out=w272:errorcluster)  [unwired: 1 in, 6 out]
            n110 = invoke class="MG17Motor" method="MoveAbsoluteEx"(reference=w286, error in=w285, "lChanID"=w284, "fAbsPosCh1"=w261, "fAbsPosCh2"=w261, "bWait"=FALSE) -> (error out=w271:errorcluster)  [unwired: 1 in, 6 out]
            n111 = invoke class="MG17Motor" method="MoveAbsoluteEx"(reference=w277, error in=w276, "lChanID"=w275, "fAbsPosCh1"=w260, "fAbsPosCh2"=w260, "bWait"=FALSE) -> (error out=w270:errorcluster)  [unwired: 1 in, 6 out]
            n112 = Merge Errors(w272, w271, w270) -> (w269:errorcluster)
          }
        }
      }
      event "InterfaceSelector": Value Change {
        n113 = event-data() -> ("NewVal"=w301:T5)  [unwired: 1 in]
        n114 = case shown="\"Force-Extension (F4)\"" w301 {
          tunnel: [T2."BasicMode" T2."PassiveMode" T2."AcquireOffsetMode" T2."AcquireSpectrumMode" T2."Force-ExtensionMode"] -> w300
          frame "Basic Operation" {
          }
          frame "Passive Mode (F1)" {
            n115 = property on="IsPassiveModeActive?" class="Bool (strict)"("Value"=TRUE ("StopOffset")) -> ()  [unwired: 2 in, 2 out]
          }
          frame "Acquire Offset (F2)" {
            n116 = property on="IsOffsetModeActive?" class="Bool (strict)"("Value"=TRUE ("StopOffset")) -> ()  [unwired: 2 in, 2 out]
          }
          frame "Acquire Spectrum (F3)" {
          }
          frame "Force-Extension (F4)" {
            n117 = property on="IsForceExtActive?" class="Bool (strict)"("Value"=TRUE ("StopOffset")) -> ()  [unwired: 2 in, 2 out]
          }
        }
        "InstrumentMode" <- w300
      }
      event "StopOffset": Value Change {
        n118 = event-data() -> ("NewVal"=w310:bool)  [unwired: 1 in, 5 out]
        n119 = case shown="True" w310 {
          frame False {
          }
          frame True {
            n120 = flat-sequence {
              frame #0 {
                n121 = Not(x="StopOffset") -> (.not. x?=→"IsOffsetModeActive?":bool)
              }
              frame #1 {
                n122 = property on="InterfaceSelector" class="TabCtl (strict)"("Value"=T5."Basic Operation" ("InterfaceSelector")) -> ()  [unwired: 2 in, 2 out]
                n123 = property on="InstrumentMode" class="Enum (strict)"("Value"=T2."BasicMode" ("InstrumentMode")) -> ()  [unwired: 2 in, 2 out]
              }
            }
          }
        }
      }
      event "StopPassiveMode": Value Change {
        n124 = event-data() -> ("NewVal"=w315:bool)  [unwired: 1 in, 5 out]
        n125 = case shown="True" w315 {
          frame False {
          }
          frame True {
            n126 = flat-sequence {
              frame #0 {
                n127 = Not(x="StopPassiveMode") -> (.not. x?=→"IsPassiveModeActive?":bool)
              }
              frame #1 {
                n128 = property on="InterfaceSelector" class="TabCtl (strict)"("Value"=T5."Basic Operation" ("InterfaceSelector")) -> ()  [unwired: 2 in, 2 out]
                n129 = property on="InstrumentMode" class="Enum (strict)"("Value"=T2."BasicMode" ("InstrumentMode")) -> ()  [unwired: 2 in, 2 out]
              }
            }
          }
        }
      }
      event "StopForceExtension": Value Change {
        n130 = event-data() -> ("NewVal"=w320:bool)  [unwired: 1 in, 5 out]
        n131 = case shown="True" w320 {
          frame False {
          }
          frame True {
            n132 = flat-sequence {
              frame #0 {
                n133 = Not(x="StopForceExtension") -> (.not. x?=→"IsForceExtActive?":bool)
              }
              frame #1 {
                n134 = property on="InterfaceSelector" class="TabCtl (strict)"("Value"=T5."Basic Operation" ("InterfaceSelector")) -> ()  [unwired: 2 in, 2 out]
                n135 = property on="InstrumentMode" class="Enum (strict)"("Value"=T2."BasicMode" ("InstrumentMode")) -> ()  [unwired: 2 in, 2 out]
              }
            }
          }
        }
      }
      event "Stop": Value Change {
        n136 = event-data() -> ()  [unwired: 1 in, 1 out]
        n137 = property on="InstrumentMode" class="Enum (strict)"("Value"=T2."Shutdown") -> ()  [unwired: 2 in, 2 out]
      }
    }
  }
  n138 = while {
    shift-right: [w330] -> _
    shift-left: T2."InitializeJoystick" -> [w329]
    shift-right: [w344] -> _
    shift-left: _ -> [w337]
    shift-right: [w341] -> _
    shift-left: _ -> [w343]
    shift-right: [w342] -> _
    shift-left: _ -> [w340]
    shift-right: [w339] -> _
    shift-left: _ -> [w338]
    shift-right: [w336] -> _
    shift-left: _ -> [w333]
    shift-right: [w334] -> _
    shift-left: _ -> [w335]
    i -> [w328]
    stop <- w331 stop-if-true
    # "Motor Control Loop"
    # ">Joystick Offset>"
    # ">RelJoyPos>"
    # ">XYZ Motor Ref>"
    # ">Error>"
    # ">Joystick Task ID>"
    # ">Joystick Buttons>"
    n139 = Wait (ms)(milliseconds to wait="MotorLoopDelay") -> ()  [unwired: 1 out]
    n140 = case shown="\"BasicMode\"" w329 {
      tunnel: [w352 _ w455 w547 w554 w561 w568 _] -> w344
      tunnel: [w350 w370 w444 w551 w558 w565 w572 w591] -> w330
      tunnel: w343 -> [w349 w418 w457 w550 w557 w564 w571 w576]
      tunnel: [w351 _ w456 w545 w552 w559 w566 _] -> w342
      tunnel: [w348 w369 w448 w550 w557 w564 w571 w573] -> w341
      tunnel: w340 -> [_ _ w437 w545 w552 w559 w566 w575]
      tunnel: [_ _ w443 w546 w553 w560 w567 _] -> w339
      tunnel: w338 -> [_ _ w442 w546 w553 w560 w567 _]
      tunnel: w337 -> [_ _ w453 w547 w554 w561 w568 _]
      tunnel: [_ _ _ _ _ _ _ TRUE ("status")] -> w331
      tunnel: [_ w417 w447 w549 w556 w563 w570 _] -> w336
      tunnel: w333 -> [_ _ w447 w549 w556 w563 w570 w577]
      tunnel: [_ _ w445 w548 w555 w562 w569 _] -> w334
      tunnel: w335 -> [_ _ w454 w548 w555 w562 w569 _]
      tunnel: w328 -> [_ _ w440 _ _ _ _ _]
      frame "InitializeJoystick" {
        # "Initialize Joystick and Shutter Controls"
        n141 = flat-sequence {
          tunnel: w349 -> [w354]
          tunnel: [w353] -> w347
          tunnel: w347 -> [w359]
          tunnel: [w358] -> w346
          tunnel: [w357] -> w345
          tunnel: [w365] -> w352
          tunnel: [w361] -> w351
          tunnel: [T2."InitializeMotors"] -> w350
          tunnel: w346 -> [w362]
          tunnel: [w362] -> w348
          tunnel: w345 -> [w361]
          frame #0 {
            n142 = call <vilib>:"Query Input Devices.vi"("error in (no error)"=w354) -> ("error out"=w353:errorcluster, "joystick info"=→"joystick info":T1)  [unwired: 7 in, 2 out]
            n143 = Wait (ms)(milliseconds to wait=u32 100) -> ()  [unwired: 1 out]
          }
          frame #1 {
            n144 = call <vilib>:"Initialize Joystick.vi"("error in (no error)"=w359, "device index"=1) -> ("error out"=w358:errorcluster, "device ID"=w357:refnum<k1>)  [unwired: 8 in]
          }
          frame #2 {
            n145 = property on="JoystOffset" class="Clust (strict)"() -> ("Value"=w364:T3)  [unwired: 2 in, 2 out]
            n146 = Bundle By Name(cluster=w364, "XOffset"=-99999, "YOffset"=-99999, "ZOffset"=-99999) -> (w365:T3)
          }
        }
      }
      frame "InitializeMotors" {
        w370 = T2."BasicMode"
        w422 = 83829794  # Z Axis Controller ID
        w428 = 83829822  # Y Axis Controller ID
        w434 = 83829798  # X Axis Controller ID
        n147 = property on="IsActive?" class="Bool (strict)"(error in=w418, "Value"=FALSE ("IsYMotorActive?")) -> (error out=w429:errorcluster)  [unwired: 1 in, 1 out]
        n148 = property on="IsActive?" class="Bool (strict)"(error in=w418, "Value"=FALSE ("IsYMotorActive?")) -> (error out=w435:errorcluster)  [unwired: 1 in, 1 out]
        n149 = property on="IsActive?" class="Bool (strict)"(error in=w418, "Value"=FALSE ("IsYMotorActive?")) -> (error out=w423:errorcluster)  [unwired: 1 in, 1 out]
        n150 = call "s_InitializeMotor.vi"("Error In"=w429, "Servo Controller  ID"=w428, "Motor Reference In"="YMotorRef") -> ("Error Out"=w430:errorcluster, "Motor Reference"=w412:refnum<k7>)
        n151 = call "s_InitializeMotor.vi"("Error In"=w435, "Servo Controller  ID"=w434, "Motor Reference In"="XMotorRef") -> ("Error Out"=w436:errorcluster, "Motor Reference"=w416:refnum<k7>)
        n152 = call "s_InitializeMotor.vi"("Error In"=w423, "Servo Controller  ID"=w422, "Motor Reference In"="ZMotorRef") -> ("Error Out"=w424:errorcluster, "Motor Reference"=w409:refnum<k7>)
        n153 = property on="IsActive?" class="Bool (strict)"(error in=w430, "Value"=TRUE ("IsYMotorActive?")) -> (error out=w411:errorcluster)  [unwired: 1 in, 1 out]
        n154 = Unbundle By Name("Motor Limits") -> ("XMin"=w376:sgl, "XMax"=w375:sgl, "YMin"=w374:sgl, "YMax"=w373:sgl, "ZMin"=w372:sgl, "ZMax"=w371:sgl)
        n155 = property on="IsActive?" class="Bool (strict)"(error in=w436, "Value"=TRUE ("IsYMotorActive?")) -> (error out=w414:errorcluster)  [unwired: 1 in, 1 out]
        n156 = property on="IsActive?" class="Bool (strict)"(error in=w424, "Value"=TRUE ("IsYMotorActive?")) -> (error out=w408:errorcluster)  [unwired: 1 in, 1 out]
        n157 = invoke class="MG17Motor" method="SetStageAxisInfo"(reference=w416, error in=w414, "lChanID"=0, "fMinPos"=w376, "fMaxPos"=w375, "lUnits"=1, "fPitch"=sgl 1.0, "lDirSense"=0) -> (reference out=w407:refnum<k7>, error out=w406:errorcluster, "lChanID"=w405:i32)  [unwired: 1 in, 6 out]
        n158 = invoke class="MG17Motor" method="SetStageAxisInfo"(reference=w412, error in=w411, "lChanID"=0, "fMinPos"=w374, "fMaxPos"=w373, "lUnits"=1, "fPitch"=sgl 1.0, "lDirSense"=0) -> (reference out=w399:refnum<k7>, error out=w398:errorcluster, "lChanID"=w397:i32)  [unwired: 1 in, 6 out]
        n159 = invoke class="MG17Motor" method="SetStageAxisInfo"(reference=w409, error in=w408, "lChanID"=0, "fMinPos"=w372, "fMaxPos"=w371, "lUnits"=1, "fPitch"=sgl 1.0, "lDirSense"=0) -> (reference out=w394:refnum<k7>, error out=w393:errorcluster, "lChanID"=w392:i32)  [unwired: 1 in, 6 out]
        n160 = invoke class="MG17Motor" method="GetPosition_Position"(reference=w399, error in=w398, "lChanID"=w397) -> (reference out=w391:refnum<k7>, error out=w401:errorcluster, "GetPosition_Position"=w400:sgl)  [unwired: 1 in, 1 out]
        n161 = invoke class="MG17Motor" method="GetPosition_Position"(reference=w394, error in=w393, "lChanID"=w392) -> (reference out=w390:refnum<k7>, error out=w396:errorcluster, "GetPosition_Position"=w395:sgl)  [unwired: 1 in, 1 out]
        n162 = invoke class="MG17Motor" method="GetPosition_Position"(reference=w407, error in=w406, "lChanID"=w405) -> (reference out=w404:refnum<k7>, error out=w403:errorcluster, "GetPosition_Position"=w402:sgl)  [unwired: 1 in, 1 out]
        n163 = property on="Pos (mm)" class="DigNum (strict)"(error in=w401, "Value"=w400) -> (error out=w389:errorcluster)  [unwired: 1 in, 1 out]
        n164 = property on="Pos (mm)" class="DigNum (strict)"(error in=w396, "Value"=w395) -> (error out=w387:errorcluster)  [unwired: 1 in, 1 out]
        n165 = property on="Pos (mm)" class="DigNum (strict)"(error in=w403, "Value"=w402) -> (error out=w388:errorcluster)  [unwired: 1 in, 1 out]
        n166 = Bundle("Motor Reference"=w404, "Motor Reference"=w391, "Motor Reference"=w390) -> (w417:T14)  [unwired: 1 in]
        n167 = Merge Errors(w388, w389, w387) -> (w369:errorcluster)
        n168 = property on="InstrumentMode" class="Enum (strict)"("Value"=w370) -> ()  [unwired: 2 in, 2 out]
      }
      frame "BasicMode" {
        n169 = First Call?() -> (First Call?: T/F=w439:bool)
        n170 = case shown="True" w439 {
          tunnel: [w458 w459] -> w438
          tunnel: w437 -> [w458 _]
          frame False {
          }
          frame True {
            n171 = call <vilib>:"Initialize Joystick.vi"("device index"=1) -> ("device ID"=w459:refnum<k1>)  [unwired: 9 in, 1 out]
          }
        }
        n172 = call-poly <vilib>:"Acquire Input Data.vi"("device ID"=w438, "Numeric"=w440, "error in (no error)"=w457) -> ("device ID 2"=w456:refnum<k1>, "axis info"=w452:T15, "button info"=w443:T16, "error out"=w441:errorcluster)  [unwired: 12 in, 1 out]
        n173 = call "j_GetJoystickSignal.vi"("RelJoyPos In"=w454, "NewJoystButtInfo"=w443, "NewJoystAxisInfo"=w452, "OldJoystButtInfo"=w442, "OldJoystickOffset"=w453) -> ("MoveZ"=→"Move Z":bool, "MoveXY"=→"Move XY":bool, "Joystick Offset"=w455:T3, "RelJoyPos"=w449:T4, "TalkToMotors?"=w446:bool)
        n174 = case shown="False" w446 {
          tunnel: w449 -> [w498 w502]
          tunnel: [w487 w519] -> w448
          tunnel: w447 -> [w497 w505]
          tunnel: w441 -> [w471 w504]
          tunnel: [w498 w502] -> w445
          frame False {
            # "Just Update Motor Position and Vel"
            n175 = Unbundle(w497) -> ("Motor Reference"=w496:refnum<k7>, "Motor Reference"=w489:refnum<k7>, "Motor Reference"=w488:refnum<k7>)
            n176 = property on="Pos (mm)" class="DigNum (strict)"(error in=w471) -> (error out=w479:errorcluster, "Value"=w476:sgl)  [unwired: 1 in, 1 out]
            n177 = property on="Pos (mm)" class="DigNum (strict)"(error in=w471) -> (error out=w472:errorcluster, "Value"=w469:sgl)  [unwired: 1 in, 1 out]
            n178 = property on="Pos (mm)" class="DigNum (strict)"(error in=w471) -> (error out=w480:errorcluster, "Value"=w485:sgl)  [unwired: 1 in, 1 out]
            n179 = invoke class="MG17Motor" method="GetPosition_Position"(reference=w489, error in=w479, "lChanID"=0) -> (error out=w492:errorcluster, "GetPosition_Position"=w477:sgl)  [unwired: 1 in, 2 out]
            n180 = invoke class="MG17Motor" method="GetPosition_Position"(reference=w488, error in=w472, "lChanID"=0) -> (error out=w490:errorcluster, "GetPosition_Position"=w468:sgl)  [unwired: 1 in, 2 out]
            n181 = property on="MotorLoopDelay" class="DigNum (strict)"() -> ("Value"=w464:u32)  [unwired: 2 in, 2 out]
            n182 = invoke class="MG17Motor" method="GetPosition_Position"(reference=w496, error in=w480, "lChanID"=0) -> (error out=w494:errorcluster, "GetPosition_Position"=w486:sgl)  [unwired: 1 in, 2 out]
            n183 = To Single Precision Float(number=w464) -> (single precision float=w463:sgl)
            n184 = Subtract(x=w486, y=w485) -> (x-y=w484:sgl)
            n185 = property on="Pos (mm)" class="DigNum (strict)"(error in=w492, "Value"=w477) -> (error out=w475:errorcluster)  [unwired: 1 in, 1 out]
            n186 = Subtract(x=w477, y=w476) -> (x-y=w478:sgl)
            n187 = Subtract(x=w468, y=w469) -> (x-y=w470:sgl)
            n188 = property on="Pos (mm)" class="DigNum (strict)"(error in=w490, "Value"=w468) -> (error out=w467:errorcluster)  [unwired: 1 in, 1 out]
            n189 = property on="Pos (mm)" class="DigNum (strict)"(error in=w494, "Value"=w486) -> (error out=w482:errorcluster)  [unwired: 1 in, 1 out]
            n190 = Divide(x=w463, y=sgl 1000.0) -> (x/y=w461:sgl)
            n191 = Divide(x=w484, y=w461) -> (x/y=w483:sgl)
            n192 = Divide(x=w478, y=w461) -> (x/y=w474:sgl)
            n193 = Divide(x=w470, y=w461) -> (x/y=w466:sgl)
            n194 = property on="Vel (mm/s)" class="DigNum (strict)"(error in=w482, "Value"=w483) -> (error out=w481:errorcluster)  [unwired: 1 in, 1 out]
            n195 = property on="Vel (mm/s)" class="DigNum (strict)"(error in=w475, "Value"=w474) -> (error out=w473:errorcluster)  [unwired: 1 in, 1 out]
            n196 = property on="Vel (mm/s)" class="DigNum (strict)"(error in=w467, "Value"=w466) -> (error out=w465:errorcluster)  [unwired: 1 in, 1 out]
            n197 = Merge Errors(w481, w473, w465) -> (w487:errorcluster)
          }
          frame True {
            # ">ZMotRef>"
            # ">YMotRef>"
            # ">XMotRef>"
            n198 = Unbundle By Name(w502) -> ("XRelPos"=w535:i32, "YRelPos"=w521:i32, "ZRelPos"=w506:i32)
            n199 = Unbundle(w505) -> ("Motor Reference"=w501:refnum<k7>, "Motor Reference"=w500:refnum<k7>, "Motor Reference"=w499:refnum<k7>)
            n200 = property on="Direction" class="DigNum (strict)"(error in=w504) -> (error out=w534:errorcluster, "Value"=w533:i32)  [unwired: 1 in, 1 out]
            n201 = property on="Direction" class="DigNum (strict)"(error in=w504) -> (error out=w524:errorcluster, "Value"=w523:i32)  [unwired: 1 in, 1 out]
            n202 = property on="Direction" class="DigNum (strict)"(error in=w504) -> (error out=w509:errorcluster, "Value"=w508:i32)  [unwired: 1 in, 1 out]
            n203 = property on="Move Z" class="Bool (strict)"(error in=w509) -> (error out=w517:errorcluster, "Value"=w516:bool)  [unwired: 1 in, 1 out]
            n204 = property on="Move XY" class="Bool (strict)"(error in=w534) -> (error out=w543:errorcluster, "Value"=w542:bool)  [unwired: 1 in, 1 out]
            n205 = property on="Move XY" class="Bool (strict)"(error in=w524) -> (error out=w532:errorcluster, "Value"=w531:bool)  [unwired: 1 in, 1 out]
            n206 = call "j_MotorExecute.vi"("MoveChamber?"=w542, "Axis Motor Settings"="X Motor Settings", "Error In"=w543, "JoystRelPos"=w535, "Motor's Old Direction"=w533, "Motor Reference In"=w501) -> ("Error Out"=w538:errorcluster, "Motor Position (mm)"=w537:sgl, "Motor's New Direction"=w536:i32, "Motor Velocity (mm/s)"=w539:sgl)  [unwired: 1 out]
            n207 = call "j_MotorExecute.vi"("MoveChamber?"=w531, "Axis Motor Settings"="Y Motor Settings", "Error In"=w532, "JoystRelPos"=w521, "Motor's Old Direction"=w523, "Motor Reference In"=w500) -> ("Error Out"=w527:errorcluster, "Motor Position (mm)"=w526:sgl, "Motor's New Direction"=w525:i32, "Motor Velocity (mm/s)"=w528:sgl)  [unwired: 1 out]
            n208 = call "j_MotorExecute.vi"("MoveChamber?"=w516, "Axis Motor Settings"="Z Motor Settings", "Error In"=w517, "JoystRelPos"=w506, "Motor's Old Direction"=w508, "Motor Reference In"=w499) -> ("Error Out"=w512:errorcluster, "Motor Position (mm)"=w511:sgl, "Motor's New Direction"=w510:i32, "Motor Velocity (mm/s)"=w513:sgl)  [unwired: 1 out]
            n209 = property on="Pos (mm)" class="DigNum (strict)"(error in=w538, "Value"=w537) -> (error out=w540:errorcluster)  [unwired: 1 in, 1 out]
            n210 = property on="Pos (mm)" class="DigNum (strict)"(error in=w527, "Value"=w526) -> (error out=w529:errorcluster)  [unwired: 1 in, 1 out]
            n211 = property on="Pos (mm)" class="DigNum (strict)"(error in=w512, "Value"=w511) -> (error out=w514:errorcluster)  [unwired: 1 in, 1 out]
            n212 = property on="Vel (mm/s)" class="DigNum (strict)"(error in=w540, "Value"=w539) -> (error out=w541:errorcluster)  [unwired: 1 in, 1 out]
            n213 = property on="Vel (mm/s)" class="DigNum (strict)"(error in=w529, "Value"=w528) -> (error out=w530:errorcluster)  [unwired: 1 in, 1 out]
            n214 = property on="Vel (mm/s)" class="DigNum (strict)"(error in=w514, "Value"=w513) -> (error out=w515:errorcluster)  [unwired: 1 in, 1 out]
            n215 = property on="Direction" class="DigNum (strict)"(error in=w530, "Value"=w525) -> (error out=w518:errorcluster)  [unwired: 1 in, 1 out]
            n216 = property on="Direction" class="DigNum (strict)"(error in=w541, "Value"=w536) -> (error out=w520:errorcluster)  [unwired: 1 in, 1 out]
            n217 = property on="Direction" class="DigNum (strict)"(error in=w515, "Value"=w510) -> (error out=w503:errorcluster)  [unwired: 1 in, 1 out]
            n218 = Merge Errors(w520, w518, w503) -> (w519:errorcluster)
          }
        }
        n219 = property on="InstrumentMode" class="Enum (strict)"() -> ("Value"=w444:T2)  [unwired: 2 in, 2 out]
      }
      frame "PassiveMode" {
        n220 = property on="InstrumentMode" class="Enum (strict)"() -> ("Value"=w551:T2)  [unwired: 2 in, 2 out]
      }
      frame "AcquireOffsetMode" {
        n221 = property on="InstrumentMode" class="Enum (strict)"() -> ("Value"=w558:T2)  [unwired: 2 in, 2 out]
      }
      frame "AcquireSpectrumMode" {
        n222 = property on="InstrumentMode" class="Enum (strict)"() -> ("Value"=w565:T2)  [unwired: 2 in, 2 out]
      }
      frame "Force-ExtensionMode" {
        n223 = property on="InstrumentMode" class="Enum (strict)"() -> ("Value"=w572:T2)  [unwired: 2 in, 2 out]
      }
      frame "Shutdown" {
        n224 = call-poly <vilib>:"Close Input Device.vi"("error in (no error)"=w576, "device ID"=w575) -> ("error out"=w584:errorcluster)  [unwired: 8 in]
        n225 = Unbundle(w577) -> ("Motor Reference"=w580:refnum<k7>, "Motor Reference"=w579:refnum<k7>, "Motor Reference"=w578:refnum<k7>)
        n226 = call "s_CloseMotor.vi"("Error In"=w584, "Motor Reference In"=w580) -> ("Error Out"=w589:errorcluster)
        n227 = call "s_CloseMotor.vi"("Error In"=w584, "Motor Reference In"=w579) -> ("Error Out"=w587:errorcluster)
        n228 = call "s_CloseMotor.vi"("Error In"=w584, "Motor Reference In"=w578) -> ("Error Out"=w585:errorcluster)
        n229 = property on="IsActive?" class="Bool (strict)"(error in=w589, "Value"=FALSE ("IsYMotorActive?")) -> (error out=w583:errorcluster)  [unwired: 1 in, 1 out]
        n230 = property on="IsActive?" class="Bool (strict)"(error in=w587, "Value"=FALSE ("IsYMotorActive?")) -> (error out=w582:errorcluster)  [unwired: 1 in, 1 out]
        n231 = property on="IsActive?" class="Bool (strict)"(error in=w585, "Value"=FALSE ("IsYMotorActive?")) -> (error out=w581:errorcluster)  [unwired: 1 in, 1 out]
        n232 = Merge Errors(w583, w582, w581) -> (w574:errorcluster)
        n233 = property on="InstrumentMode" class="Enum (strict)"(error in=w574) -> (error out=w573:errorcluster, "Value"=w591:T2)  [unwired: 1 in, 1 out]
      }
    }
  }
